vi "Update Data sub_ UT.vi"(8 "error in (no error)":errorcluster, 10 "LVData":T1, 11 "TableLogger_SQLite_Actor in":refnum<class "TableLogger_SQLite_Actor.lvclass">) -> (0 "error out":errorcluster, 2 "Update?T":bool, 3 "TableLogger_SQLite_Actor out":refnum<class "TableLogger_SQLite_Actor.lvclass">)   [LabVIEW 2014, in "TableLogger_SQLite_Actor.lvlib" / "TableLogger_SQLite_Actor.lvclass"]
uses:
  TableLogger_SQLite_Actor.lvclass
  TableLogger_SQLite_Actor.lvclass/TableLogger_SQLite_Actor.ctl
  <vilib>/drjdpowell/SQLite Library/SQL Connection/Execute SQL.vi
  <vilib>/drjdpowell/SQLite Library/SQLite.lvlib
  <vilib>/drjdpowell/SQLite Library/SQL Connection/Connection.lvclass
  TableLogger_Actor/TableLogger_Actor/TableLogger_Actor.lvclass
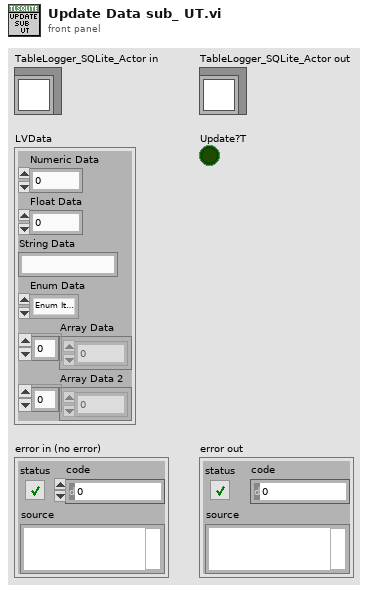
[diagram p1: front panel]
types:
  T1 = cluster{"Numeric Data":i32, "Float Data":dbl, "String Data":string, "Enum Data":enum16{"Enum Item 1", "Enum Item 2"}, "Array Data":i32[], "Array Data 2":i32[]}
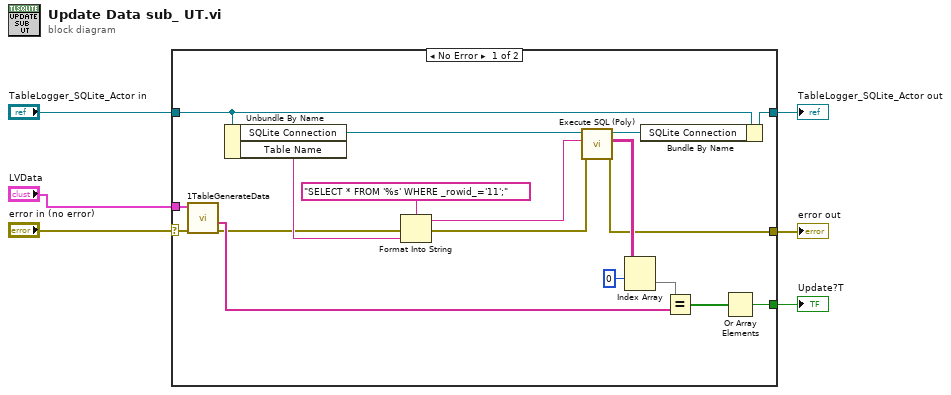
[diagram p0: block diagram]
diagram:
  n1 = case shown="No Error" "error in (no error)" {
    selector: "error in (no error)" -> [w20 w26]
    tunnel: [w24 w25] -> w6
    tunnel: "TableLogger_SQLite_Actor in" -> [w23 w25]
    tunnel: [w7 _] -> w3
    tunnel: "LVData" -> [w14 _]
    tunnel: [w12 w26] -> w1
    frame No Error {
      n2 = call "1TableGenerateData.vi"("error in (no error)"=w20, "Cluster Variant"=w14) -> ("error out"=w8:errorcluster, "Data"=w18:string[])  [unwired: 5 in, 3 out]
      n3 = Unbundle By Name(w23) -> ("SQLite Connection"=w11:refnum<class "Connection.lvclass">, "Table Name"=w13:string)
      n4 = Format Into String(format string="SELECT * FROM '%s' WHERE _rowid_='11';" ("SQL"), error in=w8, w13) -> (resulting string=w9:string, error out=w21:errorcluster)  [unwired: 1 in]
      n5 = call-poly <vilib>:"Execute SQL (Poly).vi"("error in (no error)"=w21, "SQL"=w9, "SQLite Connection in"=w11) -> ("error out"=w12:errorcluster, "Result Set"=w15:string[][], "SQLite Connection"=w22:refnum<class "Connection.lvclass">)  [unwired: 5 in, 1 out]
      n6 = Index Array(array=w15, index (row)=0) -> (element=w17:string[])  [unwired: 1 in]
      n7 = Bundle By Name(cluster=w23, "SQLite Connection"=w22) -> (w24:refnum<class "TableLogger_SQLite_Actor.lvclass">)
      n8 = Equal?(x=w17, y=w18) -> (x = y?=w19:bool[])
      n9 = Or Array Elements(Boolean array=w19) -> (logical OR=w7:bool)
    }
    frame Error {
    }
  }
  "Update?T" <- w3
  "TableLogger_SQLite_Actor out" <- w6
  "error out" <- w1
